vi "SurveyAnalyzation.vi"() -> ()   [LabVIEW 2025]
uses:
  Controls/Map.HowSafe.ctl
  Controls/Map.HowComfortable.ctl
  Controls/Map.HowDistracting.ctl
  Controls/Map.HowEasy.ctl
  Controls/Map.EasyBalance.ctl
  Controls/Map.HowPrecisely.ctl
  Controls/Map.HowIntuitive.ctl
  Controls/Map.HowFocussed.ctl
  Controls/Map.LookAway.ctl
  Controls/Map.HowEffortless.ctl
  Controls/Map.HowConfident.ctl
  Controls/Map.DontInterfere.ctl
  Controls/Map.Enjoyment.ctl
  Controls/Likert.Results.ctl
  <vilib>/Analysis/baseanly.llb/Mean (DBL).vi
  <vilib>/Utility/error.llb/Trim Whitespace One-Sided.vi
  <vilib>/Utility/file.llb/Write Delimited Spreadsheet (string).vi
  <vilib>/Analysis/NI_AALBase.lvlib
panel:
  out "std.dev.Ages":dbl format="%0.2f"
  out "Interfere.Analog.Mean":dbl
  out "Interfere.Buttons.Mean":dbl
  out "Interfere.Indirect.Touch.Mean":dbl
  out "Enjoyment.Analog.Mean":dbl
  out "Enjoyment.Buttons.Mean":dbl
  out "Enjoyment.Direct.Touch.Mean":dbl
  out "Focussed.Analog.Mean":dbl
  out "Focussed.Buttons.Mean":dbl
  out "Focussed.Indirect.Touch.Mean":dbl
  out "Effortless.Analog.Mean":dbl
  out "Effortless.Buttons.Mean":dbl
  out "Effortless.Indirect.Touch.Mean":dbl
  out "Easy.Analog.Mean":dbl
  out "Easy.Buttons.Mean":dbl
  out "Easy.Indirect.Touch.Mean":dbl
  out "Precise.Analog.Mean":dbl
  out "Precise.Buttons.Mean":dbl
  out "Precise.Indirect.Touch.Mean":dbl
  out "Look.Away.Direct.Touch.Mean":dbl
  out "Confidence.Direct.Touch.Mean":dbl
  out "Intuitive.Direct.Touch.Mean":dbl
  out "Easy.Balance.Direct.Touch.Mean":dbl
  out "Map.Enjoyment":T1
  out "Map.DontInterfere":T2
  out "Map.HowConfident":T3
  out "Map.HowEffortless":T4
  out "Map.LookAway":T5
  out "Map.HowFocussed":T6
  out "Map.HowIntuitive":T7
  out "Map.HowPrecisely":T8
  out "Map.EasyBalance":T9
  out "Map.HowEasy":T10
  out "Map.HowDistracting":T11
  out "Distracting.Direct.Touch.Mean":dbl
  out "Which input method preferred?":map{string, i32}(c390)
  out "Which input method quickest?":map{string, i32}(c390)
  out "Which input method most accurately?":map{string, i32}(c390)
  out "Which input method safest using?":map{string, i32}(c390)
  out "Which input method easiest to use?":map{string, i32}(c390)
  out "Which input method best overall?":map{string, i32}(c390)
  out "Comfortable.Analog.Mean":dbl
  out "Comfortable.Buttons.Mean":dbl
  out "Comfortable.Direct.Touch.Mean":dbl
  out "Comfortable.Indirect.Touch.Mean":dbl
  out "Safe.Indirect.Touch.Mean":dbl
  out "Safe.Direct.Touch.Mean":dbl
  out "Safe.Buttons.Mean":dbl
  out "Safe.Analog.Mean":dbl
  out "How comfortable?":T12
  out "How safe?":T13
  out "How did you use a smartphone?":map{string, i32}(c390)
  out "Environment":map{string, i32}(c390)
  out "What did you do?":map{string, i32}(c390)
  out "Smartphone usage":map{string, i32}(c390)
  out "Which type of bicycle?":map{string, i32}(c390)
  out "How often ride a bicycle?":map{string, i32}(c390)
  out "Genders":map{string, i32}(c390)
  out "Mean.Ages":dbl format="%0.2f"
  out "Ages":i32[](array[numeric])
  out "array":string[][](array[string])
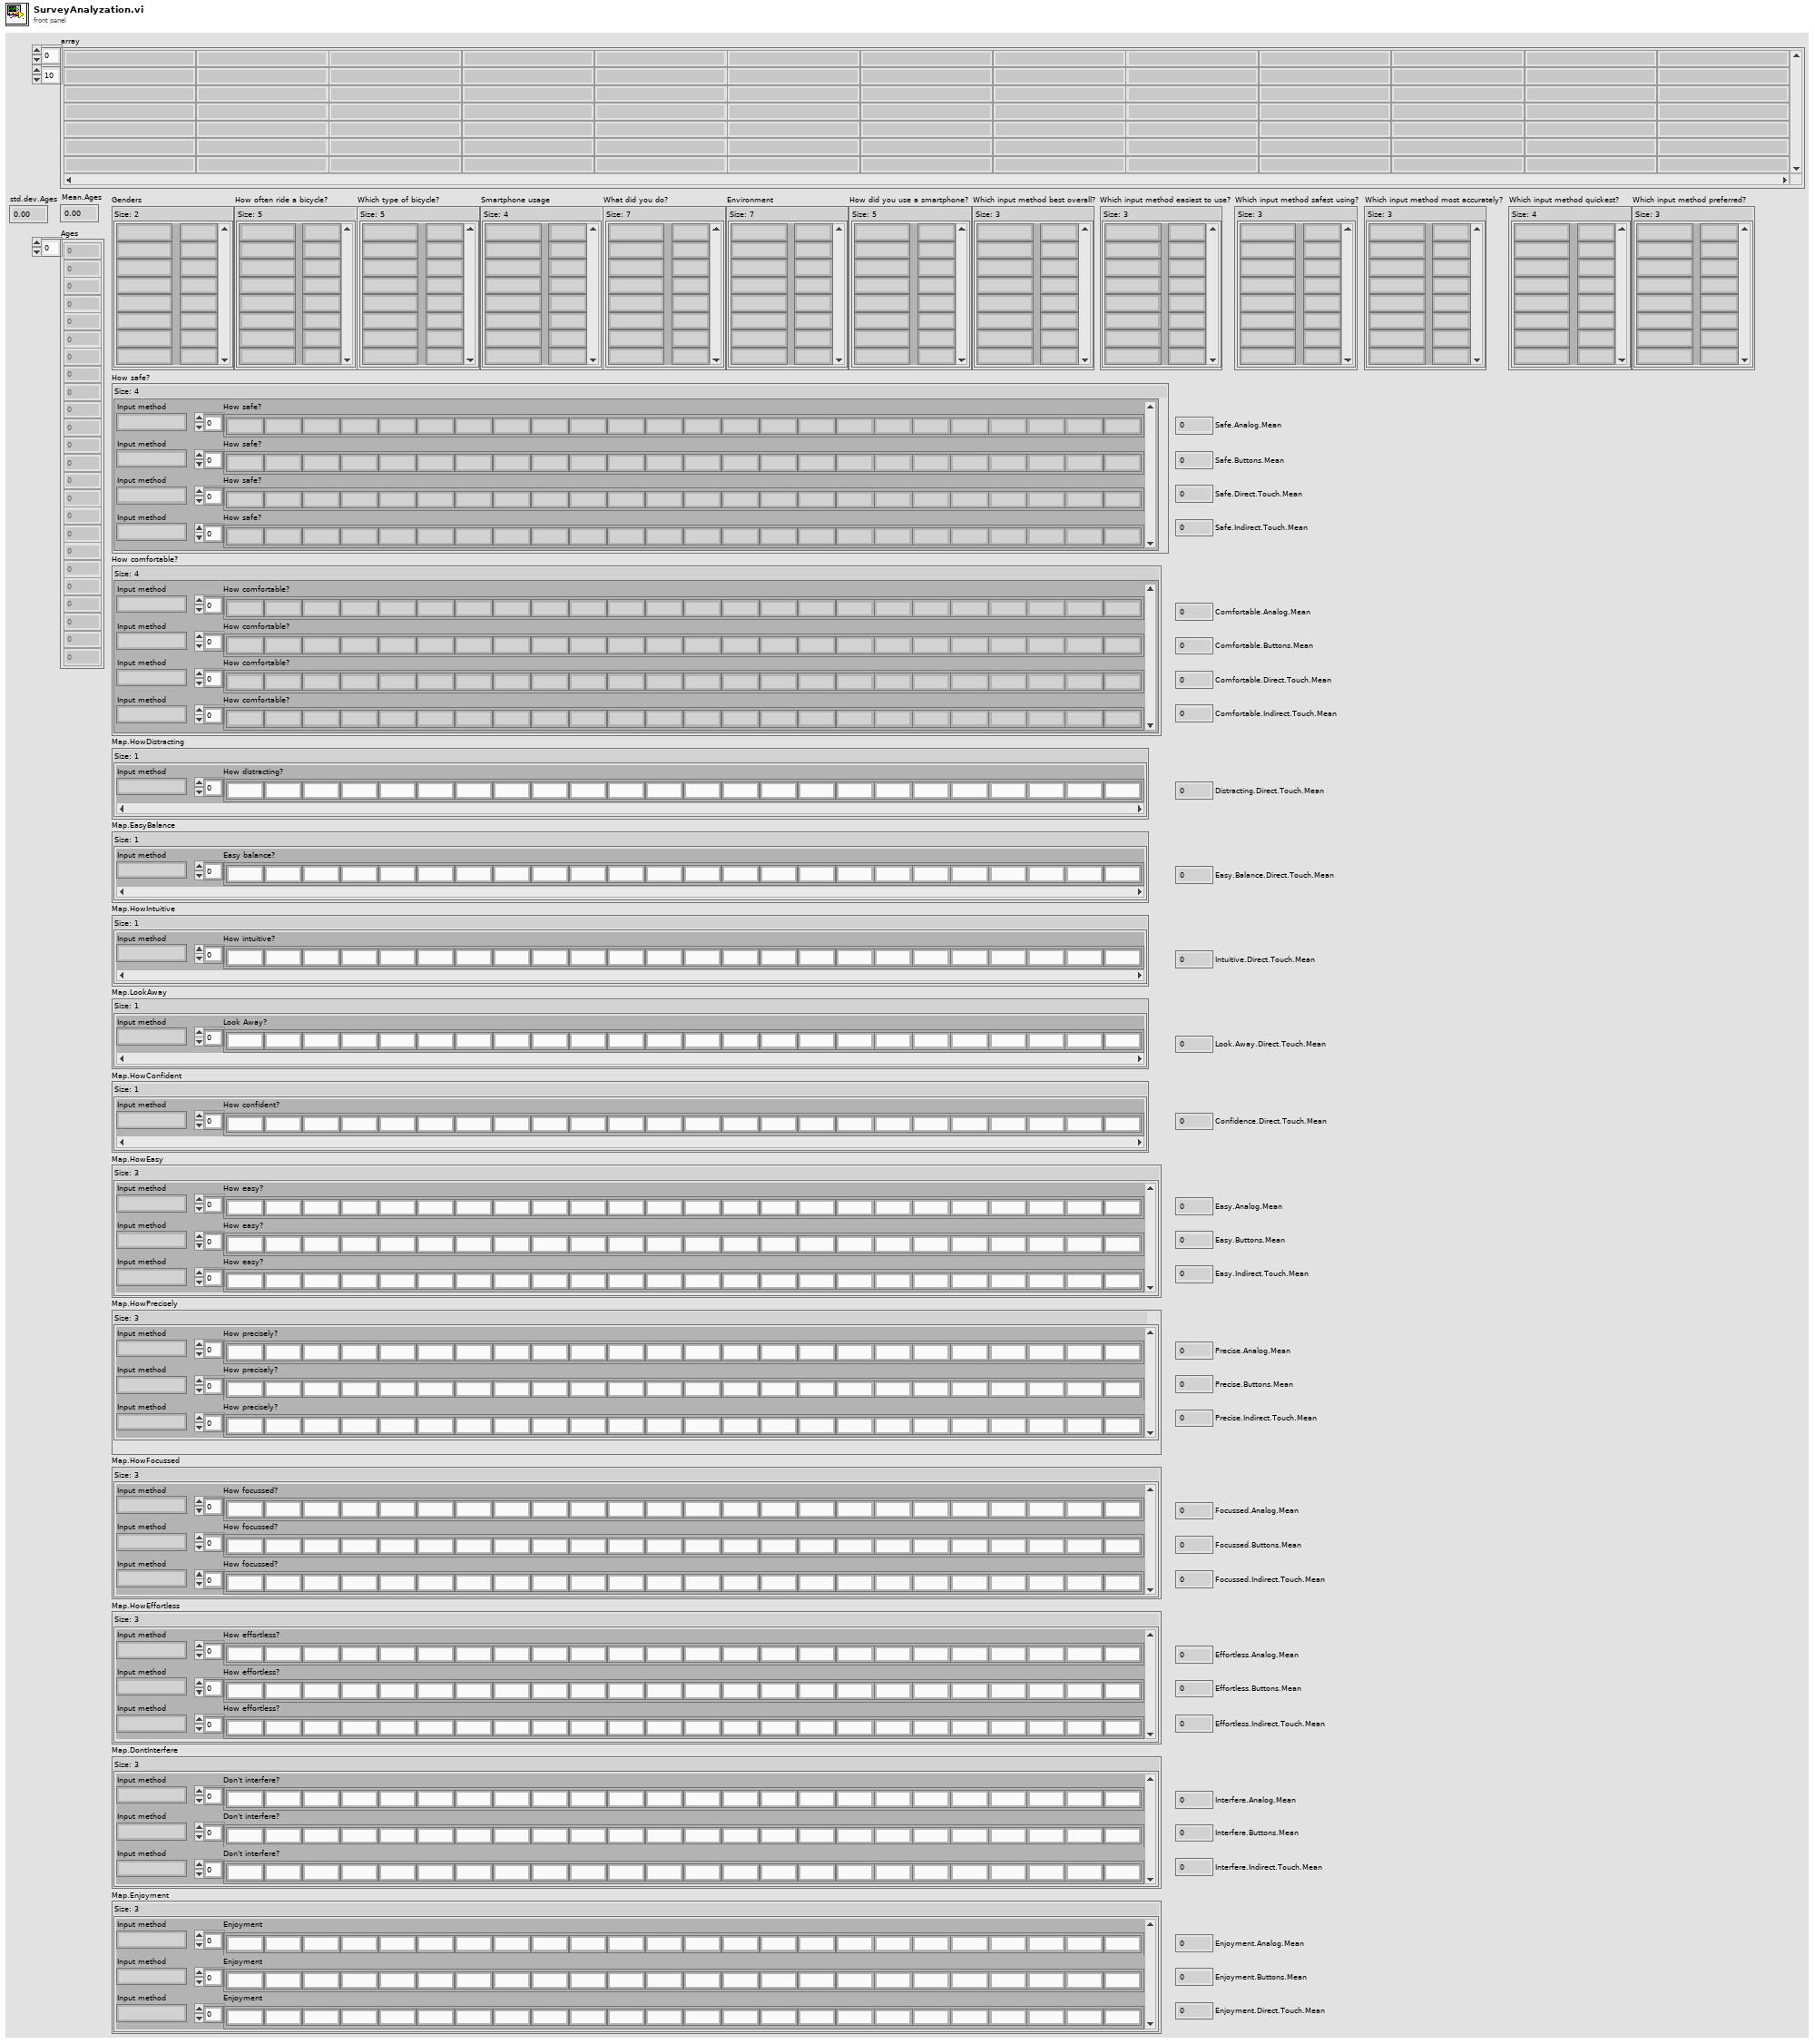
[diagram p1: front panel]
types:
  T1 = typedef "Map.Enjoyment.ctl" = map{string, i32[]}
  T2 = typedef "Map.DontInterfere.ctl" = map{string, i32[]}
  T3 = typedef "Map.HowConfident.ctl" = map{string, i32[]}
  T4 = typedef "Map.HowEffortless.ctl" = map{string, i32[]}
  T5 = typedef "Map.LookAway.ctl" = map{string, i32[]}
  T6 = typedef "Map.HowFocussed.ctl" = map{string, i32[]}
  T7 = typedef "Map.HowIntuitive.ctl" = map{string, i32[]}
  T8 = typedef "Map.HowPrecisely.ctl" = map{string, i32[]}
  T9 = typedef "Map.EasyBalance.ctl" = map{string, i32[]}
  T10 = typedef "Map.HowEasy.ctl" = map{string, i32[]}
  T11 = typedef "Map.HowDistracting.ctl" = map{string, i32[]}
  T12 = typedef "Map.HowComfortable.ctl" = map{string, i32[]}
  T13 = typedef "Map.HowSafe.ctl" = map{string, i32[]}
  T14 = typedef "Likert.Results.ctl" = cluster{"Map.HowSafe":T13, "Map.HowComfortable":T12, "Map.HowDistracting":T11, "Map.HowEasy":T10, "Map.EasyBalance":T9, "Map.HowPrecisely":T8, "Map.HowIntuitive":T7, "Map.HowFocussed":T6, "Map.LookAway":T5, "Map.HowEffortless":T4, "Map.HowConfident":T3, "Map.DontInterfere":T2, "Map.Enjoyment":T1}
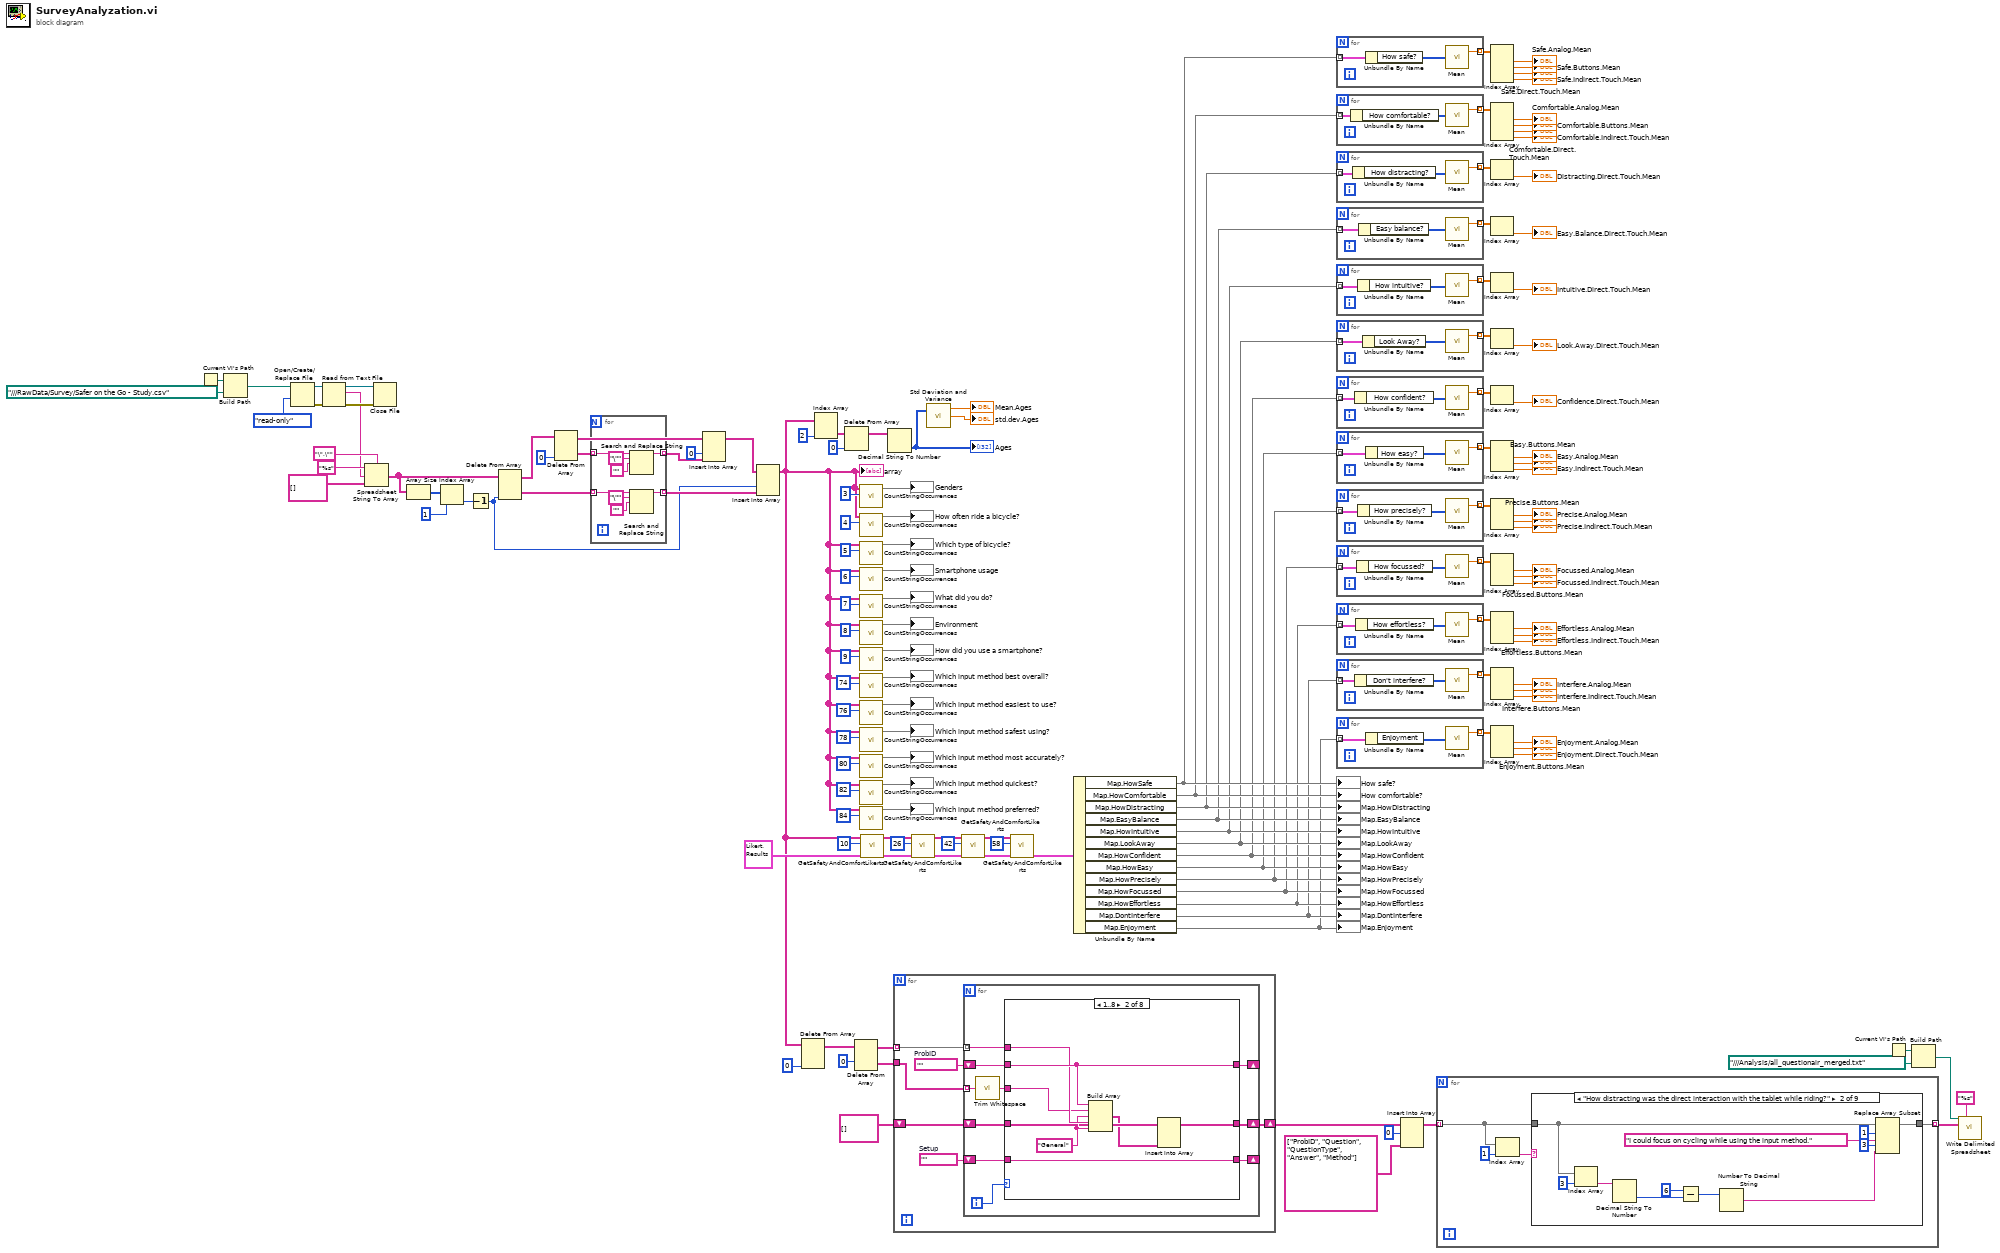
[diagram p0: block diagram]
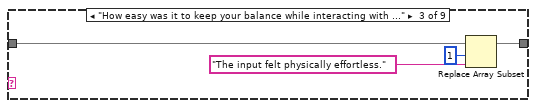
[diagram p3: hidden frame]
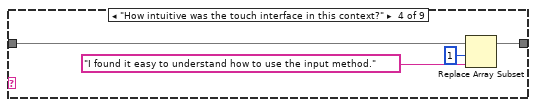
[diagram p4: hidden frame]
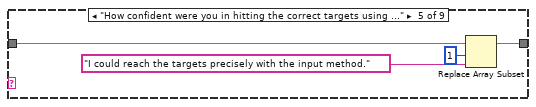
[diagram p5: hidden frame]
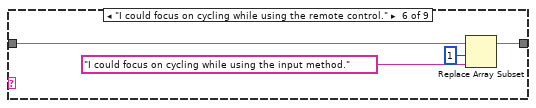
[diagram p6: hidden frame]
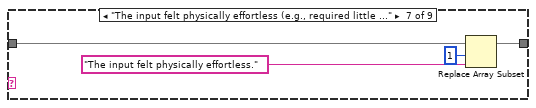
[diagram p7: hidden frame]
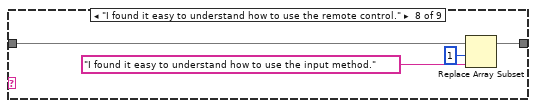
[diagram p8: hidden frame]
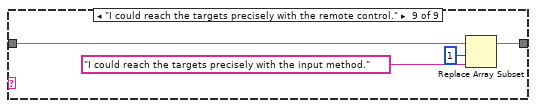
[diagram p9: hidden frame]
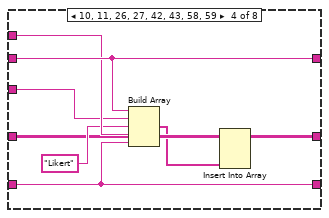
[diagram p12: hidden frame]
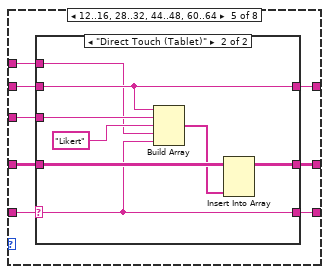
[diagram p13: hidden frame]
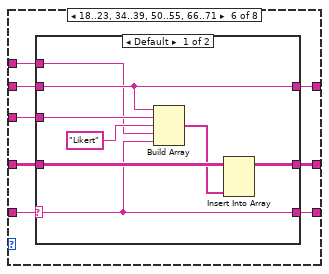
[diagram p15: hidden frame]
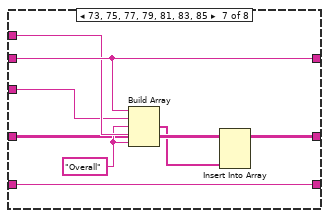
[diagram p17: hidden frame]
diagram:
  n1 = Current VI's Path() -> (path=w6:path)
  n2 = Build Path(base path=w6, name or relative path=path "../../../RawData/Survey/Safer on the Go - Study.csv") -> (appended path=w4:path)
  n3 = Open/Create/Replace File(file path (use dialog)=w4, access (0:read/write)=enum16{"read/write", "read-only", "write-only"}."read-only") -> (refnum out=w144:refnum<file>, error out=w143:errorcluster)  [unwired: 4 in, 1 out]
  n4 = Read from Text File(file (use dialog)=w144, error in=w143) -> (refnum out=w142:refnum<file>, text=w136:string, error out=w141:errorcluster)  [unwired: 2 in, 1 out]
  n5 = Spreadsheet String To Array(delimiter (Tab)="\",\"", format string="%s", spreadsheet string=w136, array type (2D Dbl)=string[][] []) -> (array=w131:string[][])
  n6 = Close File(refnum=w142, error in=w141) -> ()  [unwired: 2 out]
  n7 = Array Size(array=w131) -> (size(s)=w133:i32[])
  n8 = Index Array(array=w133, index=1) -> (element=w132:i32)
  n9 = Decrement(x=w132) -> (x-1=w123:i32)
  n10 = Delete From Array(array=w131, index (col)=w123) -> (deleted portion=w130:string[], array with subset deleted=w129:string[][])  [unwired: 2 in]
  n11 = Delete From Array(array=w129, index (col)=0 ("disabled index (col)")) -> (deleted portion=w134:string[], array with subset deleted=w128:string[][])  [unwired: 2 in]
  n12 = for {
    tunnel: w134 -> [w152] mode=indexing
    tunnel: w130 -> [w147] mode=indexing
    tunnel: [w146] -> w127 mode=indexing
    tunnel: [w145] -> w124 mode=indexing
    n13 = Search and Replace String(input string=w152, search string="\"" ("replace string (\"\")"), replace string="") -> (result string=w146:string)  [unwired: 5 in, 3 out]
    n14 = Search and Replace String(input string=w147, search string="\"" ("replace string (\"\")"), replace string="") -> (result string=w145:string)  [unwired: 5 in, 3 out]
  }
  n15 = Insert Into Array(array=w128, index (col)=0 ("disabled index (col)"), new element=w127) -> (w125:string[][])  [unwired: 1 in]
  n16 = Insert Into Array(array=w125, index (col)=w123, new element=w124) -> (w22:string[][])  [unwired: 1 in]
  "array" <- w22
  n17 = Delete From Array(array=w22, index (col)=0 ("disabled index (col)")) -> (array with subset deleted=w19:string[][])  [unwired: 2 in, 1 out]
  n18 = Index Array(array=w22, index (col)=2 ("disabled index (col)")) -> (element=w120:string[])  [unwired: 1 in]
  n19 = Delete From Array(array=w120, index=0) -> (array with subset deleted=w118:string[])  [unwired: 1 in, 1 out]
  n20 = Delete From Array(array=w19, index (row)=0) -> (deleted portion=w16:string[], array with subset deleted=w20:string[][])  [unwired: 2 in]
  n21 = call "CountStringOccurrences.vi"("Column Index"=3 ("disabled index (col)"), "Array in"=w22) -> ("String Occurences out"=→"Genders":map{string, i32})  [unwired: 9 in]
  n22 = call "CountStringOccurrences.vi"("Column Index"=4 ("disabled index (col)"), "Array in"=w22) -> ("String Occurences out"=→"How often ride a bicycle?":map{string, i32})  [unwired: 9 in]
  n23 = call "CountStringOccurrences.vi"("Column Index"=5 ("disabled index (col)"), "Array in"=w22) -> ("String Occurences out"=→"Which type of bicycle?":map{string, i32})  [unwired: 9 in]
  n24 = call "CountStringOccurrences.vi"("Column Index"=6 ("disabled index (col)"), "Array in"=w22) -> ("String Occurences out"=→"Smartphone usage":map{string, i32})  [unwired: 9 in]
  n25 = call "CountStringOccurrences.vi"("Column Index"=7 ("disabled index (col)"), "Array in"=w22) -> ("String Occurences out"=→"What did you do?":map{string, i32})  [unwired: 9 in]
  n26 = call "CountStringOccurrences.vi"("Column Index"=8 ("disabled index (col)"), "Array in"=w22) -> ("String Occurences out"=→"Environment":map{string, i32})  [unwired: 9 in]
  n27 = call "CountStringOccurrences.vi"("Column Index"=9 ("disabled index (col)"), "Array in"=w22) -> ("String Occurences out"=→"How did you use a smartphone?":map{string, i32})  [unwired: 9 in]
  n28 = call "CountStringOccurrences.vi"("Column Index"=74 ("disabled index (col)"), "Array in"=w22) -> ("String Occurences out"=→"Which input method best overall?":map{string, i32})  [unwired: 9 in]
  n29 = call "CountStringOccurrences.vi"("Column Index"=76 ("disabled index (col)"), "Array in"=w22) -> ("String Occurences out"=→"Which input method easiest to use?":map{string, i32})  [unwired: 9 in]
  n30 = call "CountStringOccurrences.vi"("Column Index"=78 ("disabled index (col)"), "Array in"=w22) -> ("String Occurences out"=→"Which input method safest using?":map{string, i32})  [unwired: 9 in]
  n31 = call "CountStringOccurrences.vi"("Column Index"=80 ("disabled index (col)"), "Array in"=w22) -> ("String Occurences out"=→"Which input method most accurately?":map{string, i32})  [unwired: 9 in]
  n32 = call "CountStringOccurrences.vi"("Column Index"=82 ("disabled index (col)"), "Array in"=w22) -> ("String Occurences out"=→"Which input method quickest?":map{string, i32})  [unwired: 9 in]
  n33 = call "CountStringOccurrences.vi"("Column Index"=84 ("disabled index (col)"), "Array in"=w22) -> ("String Occurences out"=→"Which input method preferred?":map{string, i32})  [unwired: 9 in]
  n34 = call "GetSafetyAndComfortLikerts.vi"("Likert.Results"=T14 {"Map.HowSafe"={}, "Map.HowComfortable"={}, "Map.HowDistracting"={}, "Map.HowEasy"={}, "Map.EasyBalance"={}, "Map.HowPrecisely"={}, "Map.HowIntuitive"={}, "Map.HowFocussed"={}, "Map.LookAway"={}, "Map.HowEffortless"={}, "Map.HowConfident"={}, "Map.DontInterfere"={}, "Map.Enjoyment"={}}, "Column index in"=10 ("disabled index (col)"), "Data array in"=w22) -> ("Likert.Results.out"=w73:T14, "Data array out"=w101:string[][])  [unwired: 7 in]
  n35 = Decimal String To Number(string=w118) -> (number=w9:i32[])  [unwired: 2 in, 1 out]
  "Ages" <- w9
  n36 = for {
    tunnel: w20 -> [w158] mode=indexing
    shift-right: [w155] -> w14
    shift-left: string[][] [] -> [w156]
    tunnel: w16 -> [w154]
    w153 = ""  # Setup
    w157 = ""  # ProbID
    n37 = for {
      tunnel: w158 -> [w167] mode=indexing
      shift-right: [w166] -> _
      shift-left: w157 -> [w165]
      shift-right: [w163] -> w155
      shift-left: w156 -> [w164]
      tunnel: w154 -> [w160] mode=indexing
      shift-right: [w162] -> _
      shift-left: w153 -> [w161]
      i -> [w168]
      n38 = call <vilib>:"Trim Whitespace.vi"("string"=w160) -> ("trimmed string"=w159:string)  [unwired: 1 in]
      n39 = case shown="1..8" w168 {
        tunnel: w167 -> [w171 w178 w182 w189 w191 w210 w235 _]
        tunnel: [w171 w179 w181 w190 w194 w213 w236 w239] -> w166
        tunnel: w165 -> [_ w179 w181 w190 w195 w214 w236 w239]
        tunnel: w164 -> [w170 w176 w180 w187 w197 w216 w233 w238]
        tunnel: [w170 w174 w180 w185 w196 w215 w231 w238] -> w163
        tunnel: w159 -> [_ w173 _ w184 w192 w211 w230 _]
        tunnel: [w169 w172 w182 w183 w193 w212 w229 w237] -> w162
        tunnel: w161 -> [w169 w172 _ w183 w198 w217 w229 w237]
        frame 0 {
        }
        frame 1..8 {
          w177 = "General"
          n40 = Build Array(w179, w173, w177, w178, w177) -> (w175:string[])
          n41 = Insert Into Array(array=w176, new element=w175) -> (w174:string[][])  [unwired: 2 in]
        }
        frame 9, 25, 41, 57 {
        }
        frame 10, 11, 26, 27, 42, 43, 58, 59 {
          n42 = Build Array(w190, w184, "Likert", w189, w183) -> (w186:string[])
          n43 = Insert Into Array(array=w187, new element=w186) -> (w185:string[][])  [unwired: 2 in]
        }
        frame 12..16, 28..32, 44..48, 60..64 {
          n44 = case shown="\"Direct Touch (Tablet)\"" w198 {
            selector: w198 -> [w199 w203]
            tunnel: w197 -> [w201 w208]
            tunnel: [w201 w209] -> w196
            tunnel: w195 -> [w200 w207]
            tunnel: [w200 w207] -> w194
            tunnel: [w199 w203] -> w193
            tunnel: w192 -> [_ w206]
            tunnel: w191 -> [_ w204]
            frame Default {
            }
            frame "Direct Touch (Tablet)" {
              n45 = Build Array(w207, w206, "Likert" ("element"), w204, w203) -> (w202:string[])
              n46 = Insert Into Array(array=w208, new element=w202) -> (w209:string[][])  [unwired: 2 in]
            }
          }
        }
        frame 18..23, 34..39, 50..55, 66..71 {
          n47 = case shown="Default" w217 {
            selector: w217 -> [w219 w226]
            tunnel: w216 -> [w224 w228]
            tunnel: [w225 w228] -> w215
            tunnel: w214 -> [w223 w227]
            tunnel: [w223 w227] -> w213
            tunnel: [w219 w226] -> w212
            tunnel: w211 -> [w222 _]
            tunnel: w210 -> [w220 _]
            frame Default {
              n48 = Build Array(w223, w222, "Likert" ("element"), w220, w219) -> (w218:string[])
              n49 = Insert Into Array(array=w224, new element=w218) -> (w225:string[][])  [unwired: 2 in]
            }
            frame "Direct Touch (Tablet)" {
            }
          }
        }
        frame 73, 75, 77, 79, 81, 83, 85 {
          w234 = "Overall"
          n50 = Build Array(w236, w230, w234, w235, w234) -> (w232:string[])
          n51 = Insert Into Array(array=w233, new element=w232) -> (w231:string[][])  [unwired: 2 in]
        }
        frame Default {
        }
      }
    }
  }
  n52 = call "GetSafetyAndComfortLikerts.vi"("Likert.Results"=w73, "Column index in"=26, "Data array in"=w101) -> ("Likert.Results.out"=w72:T14, "Data array out"=w102:string[][])  [unwired: 7 in]
  n53 = call <vilib>:"Std Deviation and Variance.vi"("X"=w9) -> ("mean"=→"Mean.Ages":dbl, "standard deviation"=→"std.dev.Ages":dbl)  [unwired: 1 in, 1 out]
  n54 = call "GetSafetyAndComfortLikerts.vi"("Likert.Results"=w72, "Column index in"=42, "Data array in"=w102) -> ("Likert.Results.out"=w99:T14, "Data array out"=w100:string[][])  [unwired: 7 in]
  n55 = call "GetSafetyAndComfortLikerts.vi"("Likert.Results"=w99, "Column index in"=58, "Data array in"=w100) -> ("Likert.Results.out"=w70:T14)  [unwired: 7 in, 1 out]
  n56 = Unbundle By Name(w70) -> ("Map.HowSafe"=w69:T13, "Map.HowComfortable"=w66:T12, "Map.HowDistracting"=w65:T11, "Map.EasyBalance"=w56:T9, "Map.HowIntuitive"=w55:T7, "Map.LookAway"=w54:T5, "Map.HowConfident"=w53:T3, "Map.HowEasy"=w28:T10, "Map.HowPrecisely"=w27:T8, "Map.HowFocussed"=w26:T6, "Map.HowEffortless"=w25:T4, "Map.DontInterfere"=w24:T2, "Map.Enjoyment"=w23:T1)
  "How safe?" <- w69
  "How comfortable?" <- w66
  "Map.HowDistracting" <- w65
  "Map.HowEasy" <- w28
  "Map.EasyBalance" <- w56
  "Map.HowPrecisely" <- w27
  "Map.HowIntuitive" <- w55
  "Map.HowFocussed" <- w26
  "Map.LookAway" <- w54
  "Map.HowEffortless" <- w25
  "Map.HowConfident" <- w53
  "Map.DontInterfere" <- w24
  "Map.Enjoyment" <- w23
  n57 = for {
    tunnel: w69 -> [w242] mode=indexing
    tunnel: [w240] -> w95 mode=indexing
    n58 = Unbundle By Name(w242) -> ("How safe?"=w241:i32[])
    n59 = call-poly <vilib>:"Mean.vi"("X"=w241) -> ("mean"=w240:dbl)  [unwired: 1 out]
  }
  n60 = for {
    tunnel: w66 -> [w245] mode=indexing
    tunnel: [w243] -> w86 mode=indexing
    n61 = Unbundle By Name(w245) -> ("How comfortable?"=w244:i32[])
    n62 = call-poly <vilib>:"Mean.vi"("X"=w244) -> ("mean"=w243:dbl)  [unwired: 1 out]
  }
  n63 = for {
    tunnel: w65 -> [w248] mode=indexing
    tunnel: [w246] -> w68 mode=indexing
    n64 = Unbundle By Name(w248) -> ("How distracting?"=w247:i32[])
    n65 = call-poly <vilib>:"Mean.vi"("X"=w247) -> ("mean"=w246:dbl)  [unwired: 1 out]
  }
  n66 = for {
    tunnel: w56 -> [w251] mode=indexing
    tunnel: [w249] -> w63 mode=indexing
    n67 = Unbundle By Name(w251) -> ("Easy balance?"=w250:i32[])
    n68 = call-poly <vilib>:"Mean.vi"("X"=w250) -> ("mean"=w249:dbl)  [unwired: 1 out]
  }
  n69 = for {
    tunnel: w55 -> [w254] mode=indexing
    tunnel: [w252] -> w62 mode=indexing
    n70 = Unbundle By Name(w254) -> ("How intuitive?"=w253:i32[])
    n71 = call-poly <vilib>:"Mean.vi"("X"=w253) -> ("mean"=w252:dbl)  [unwired: 1 out]
  }
  n72 = for {
    tunnel: w54 -> [w257] mode=indexing
    tunnel: [w255] -> w58 mode=indexing
    n73 = Unbundle By Name(w257) -> ("Look Away?"=w256:i32[])
    n74 = call-poly <vilib>:"Mean.vi"("X"=w256) -> ("mean"=w255:dbl)  [unwired: 1 out]
  }
  n75 = for {
    tunnel: w53 -> [w260] mode=indexing
    tunnel: [w258] -> w59 mode=indexing
    n76 = Unbundle By Name(w260) -> ("How confident?"=w259:i32[])
    n77 = call-poly <vilib>:"Mean.vi"("X"=w259) -> ("mean"=w258:dbl)  [unwired: 1 out]
  }
  n78 = for {
    tunnel: w28 -> [w263] mode=indexing
    tunnel: [w261] -> w45 mode=indexing
    n79 = Unbundle By Name(w263) -> ("How easy?"=w262:i32[])
    n80 = call-poly <vilib>:"Mean.vi"("X"=w262) -> ("mean"=w261:dbl)  [unwired: 1 out]
  }
  n81 = for {
    tunnel: [w266] -> w52 mode=indexing
    tunnel: w27 -> [w265] mode=indexing
    n82 = Unbundle By Name(w265) -> ("How precisely?"=w264:i32[])
    n83 = call-poly <vilib>:"Mean.vi"("X"=w264) -> ("mean"=w266:dbl)  [unwired: 1 out]
  }
  n84 = for {
    tunnel: [w269] -> w44 mode=indexing
    tunnel: w26 -> [w267] mode=indexing
    n85 = Unbundle By Name(w267) -> ("How focussed?"=w268:i32[])
    n86 = call-poly <vilib>:"Mean.vi"("X"=w268) -> ("mean"=w269:dbl)  [unwired: 1 out]
  }
  n87 = for {
    tunnel: [w272] -> w37 mode=indexing
    tunnel: w25 -> [w270] mode=indexing
    n88 = Unbundle By Name(w270) -> ("How effortless?"=w271:i32[])
    n89 = call-poly <vilib>:"Mean.vi"("X"=w271) -> ("mean"=w272:dbl)  [unwired: 1 out]
  }
  n90 = for {
    tunnel: [w275] -> w29 mode=indexing
    tunnel: w24 -> [w273] mode=indexing
    n91 = Unbundle By Name(w273) -> ("Don't interfere?"=w274:i32[])
    n92 = call-poly <vilib>:"Mean.vi"("X"=w274) -> ("mean"=w275:dbl)  [unwired: 1 out]
  }
  n93 = for {
    tunnel: [w278] -> w36 mode=indexing
    tunnel: w23 -> [w276] mode=indexing
    n94 = Unbundle By Name(w276) -> ("Enjoyment"=w277:i32[])
    n95 = call-poly <vilib>:"Mean.vi"("X"=w277) -> ("mean"=w278:dbl)  [unwired: 1 out]
  }
  n96 = Insert Into Array(array=w14, index (row)=0, new element=string[] ["ProbID", "Question", "QuestionType", "Answer", "Method"] ("new element/subarray")) -> (w11:string[][])  [unwired: 1 in]
  n97 = for {
    tunnel: w11 -> [w279] mode=indexing
    tunnel: [w280] -> w10 mode=indexing
    n98 = Index Array(array=w279, index=1) -> (element=w281:string)
    n99 = case shown="\"How distracting was the direct interaction with the tablet while riding?\"" w281 {
      tunnel: [w283 w292 w296 w300 w304 w308 w312 w316 w320] -> w280
      tunnel: w279 -> [w283 w290 w295 w299 w303 w307 w311 w315 w319]
      frame Default {
      }
      frame "How distracting was the direct interaction with the tablet while riding?" {
        n100 = Index Array(array=w290, index=3) -> (element=w288:string)
        n101 = Decimal String To Number(string=w288) -> (number=w285:i32)  [unwired: 2 in, 1 out]
        n102 = Subtract(x=6, y=w285) -> (x-y=w287:i32)
        n103 = Number To Decimal String(number=w287) -> (decimal integer string=w286:string)  [unwired: 1 in]
        n104 = Replace Array Subset(array=w290, new element #1="I could focus on cycling while using the input method.", index #1=1 ("index"), new element #2=w286, index #2=3 ("index")) -> (w292:string[])
      }
      frame "How easy was it to keep your balance while interacting with the touchscreen?" {
        n105 = Replace Array Subset(array=w295, new element="The input felt physically effortless.", index=1) -> (w296:string[])
      }
      frame "How intuitive was the touch interface in this context?" {
        n106 = Replace Array Subset(array=w299, new element="I found it easy to understand how to use the input method.", index=1) -> (w300:string[])
      }
      frame "How confident were you in hitting the correct targets using touch input?" {
        n107 = Replace Array Subset(array=w303, new element="I could reach the targets precisely with the input method.", index=1) -> (w304:string[])
      }
      frame "I could focus on cycling while using the remote control." {
        n108 = Replace Array Subset(array=w307, new element="I could focus on cycling while using the input method.", index=1) -> (w308:string[])
      }
      frame "The input felt physically effortless (e.g., required little strength or finger movement)." {
        n109 = Replace Array Subset(array=w311, new element="The input felt physically effortless.", index=1) -> (w312:string[])
      }
      frame "I found it easy to understand how to use the remote control." {
        n110 = Replace Array Subset(array=w315, new element="I found it easy to understand how to use the input method.", index=1) -> (w316:string[])
      }
      frame "I could reach the targets precisely with the remote control." {
        n111 = Replace Array Subset(array=w319, new element="I could reach the targets precisely with the input method.", index=1) -> (w320:string[])
      }
    }
  }
  n112 = Index Array(array=w95) -> (element #1=→"Safe.Analog.Mean":dbl, element #2=→"Safe.Buttons.Mean":dbl, element #3=→"Safe.Direct.Touch.Mean":dbl, element #4=→"Safe.Indirect.Touch.Mean":dbl)  [unwired: 4 in]
  n113 = Index Array(array=w86) -> (element #1=→"Comfortable.Analog.Mean":dbl, element #2=→"Comfortable.Buttons.Mean":dbl, element #3=→"Comfortable.Direct.Touch.Mean":dbl, element #4=→"Comfortable.Indirect.Touch.Mean":dbl)  [unwired: 4 in]
  n114 = Index Array(array=w68) -> (element=→"Distracting.Direct.Touch.Mean":dbl)  [unwired: 1 in]
  n115 = Index Array(array=w63) -> (element=→"Easy.Balance.Direct.Touch.Mean":dbl)  [unwired: 1 in]
  n116 = Index Array(array=w62) -> (element=→"Intuitive.Direct.Touch.Mean":dbl)  [unwired: 1 in]
  n117 = Index Array(array=w58) -> (element=→"Look.Away.Direct.Touch.Mean":dbl)  [unwired: 1 in]
  n118 = Index Array(array=w59) -> (element=→"Confidence.Direct.Touch.Mean":dbl)  [unwired: 1 in]
  n119 = Index Array(array=w45) -> (element #1=→"Easy.Analog.Mean":dbl, element #2=→"Easy.Buttons.Mean":dbl, element #3=→"Easy.Indirect.Touch.Mean":dbl)  [unwired: 3 in]
  n120 = Index Array(array=w52) -> (element #1=→"Precise.Analog.Mean":dbl, element #2=→"Precise.Buttons.Mean":dbl, element #3=→"Precise.Indirect.Touch.Mean":dbl)  [unwired: 3 in]
  n121 = Index Array(array=w44) -> (element #1=→"Focussed.Analog.Mean":dbl, element #2=→"Focussed.Buttons.Mean":dbl, element #3=→"Focussed.Indirect.Touch.Mean":dbl)  [unwired: 3 in]
  n122 = Index Array(array=w37) -> (element #1=→"Effortless.Analog.Mean":dbl, element #2=→"Effortless.Buttons.Mean":dbl, element #3=→"Effortless.Indirect.Touch.Mean":dbl)  [unwired: 3 in]
  n123 = Index Array(array=w29) -> (element #1=→"Interfere.Analog.Mean":dbl, element #2=→"Interfere.Buttons.Mean":dbl, element #3=→"Interfere.Indirect.Touch.Mean":dbl)  [unwired: 3 in]
  n124 = Index Array(array=w36) -> (element #1=→"Enjoyment.Analog.Mean":dbl, element #2=→"Enjoyment.Buttons.Mean":dbl, element #3=→"Enjoyment.Direct.Touch.Mean":dbl)  [unwired: 3 in]
  n125 = Current VI's Path() -> (path=w3:path)
  n126 = Build Path(base path=w3, name or relative path=path "../../../Analysis/all_questionair_merged.txt") -> (appended path=w1:path)
  n127 = call-poly <vilib>:"Write Delimited Spreadsheet.vi"("file path (dialog if empty)"=w1, "format (%s)"="%s" ("format (%.3f)"), "2D data"=w10) -> ()  [unwired: 11 in, 2 out]
